vi "数据查询_仪器日志.vi"() -> ()   [LabVIEW 2016]
uses:
  <vilib>/Utility/miscctls.llb/LVRowAndColumnUnsignedTypeDef.ctl
  <vilib>/Utility/miscctls.llb/LVPointTypeDef.ctl
  <userlib>/_OpenG.lib/array/array.llb/Sort 2D Array (String)__ogtk.vi
panel:
  in  "序列号":string
  out "总共行数":i32
  in  "显示行数":i32=15
  in  "下拉列表":string(xcontrol)
  in  "导出":bool
  in  "查询":bool
  out "数据表":string[][](table)
  in  "结束日期":string="2050/01/01"
  in  "起始日期":string="2010/01/01"
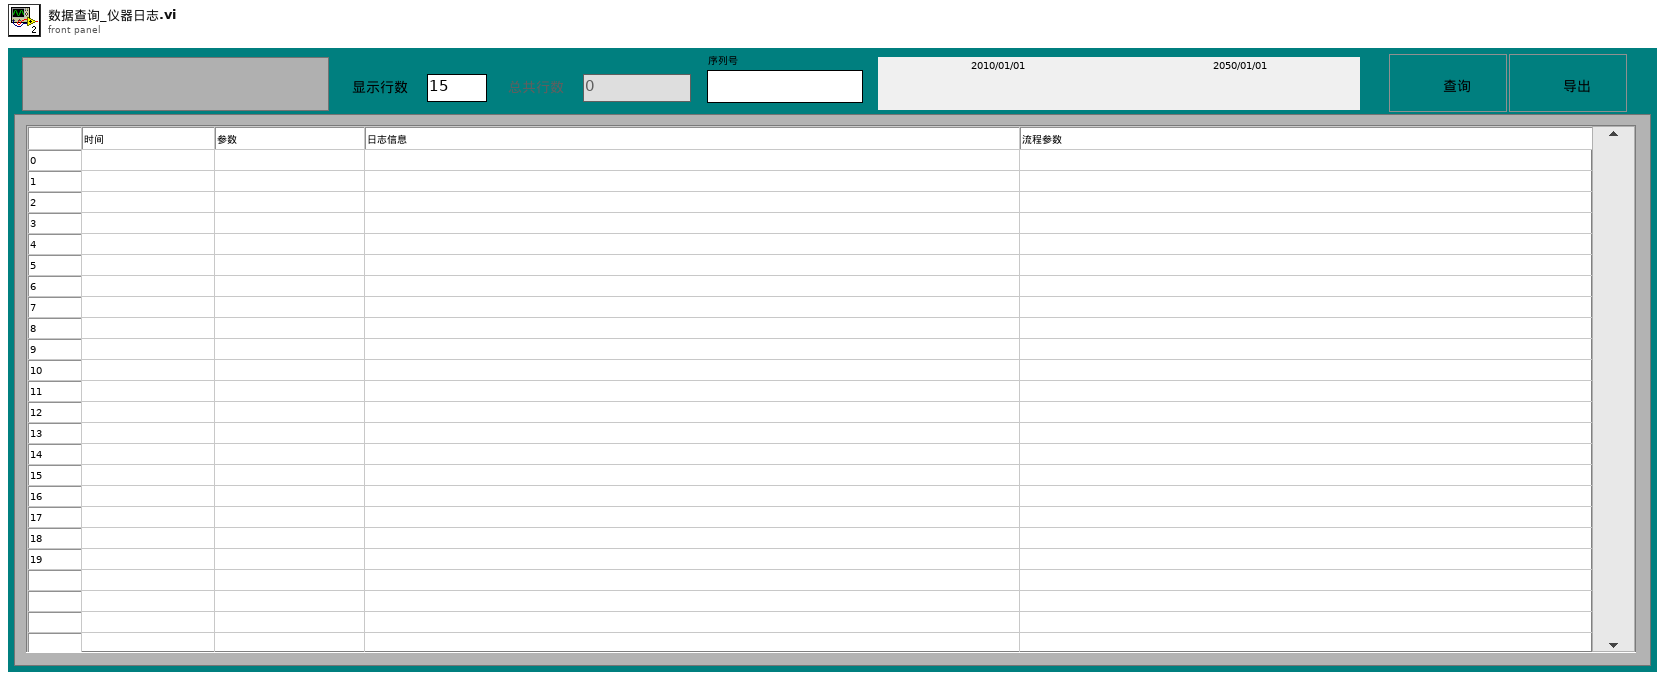
[diagram p1: front panel]
types:
  T1 = enum8{"Enabled", "Disabled", "Disabled and Grayed Out"}
  T2 = typedef "LVRowAndColumnUnsignedTypeDef.ctl" = cluster{"Row":u32, "Column":u32}
  T3 = typedef "LVPointTypeDef.ctl" = cluster{"Horizontal":i16, "Vertical":i16}
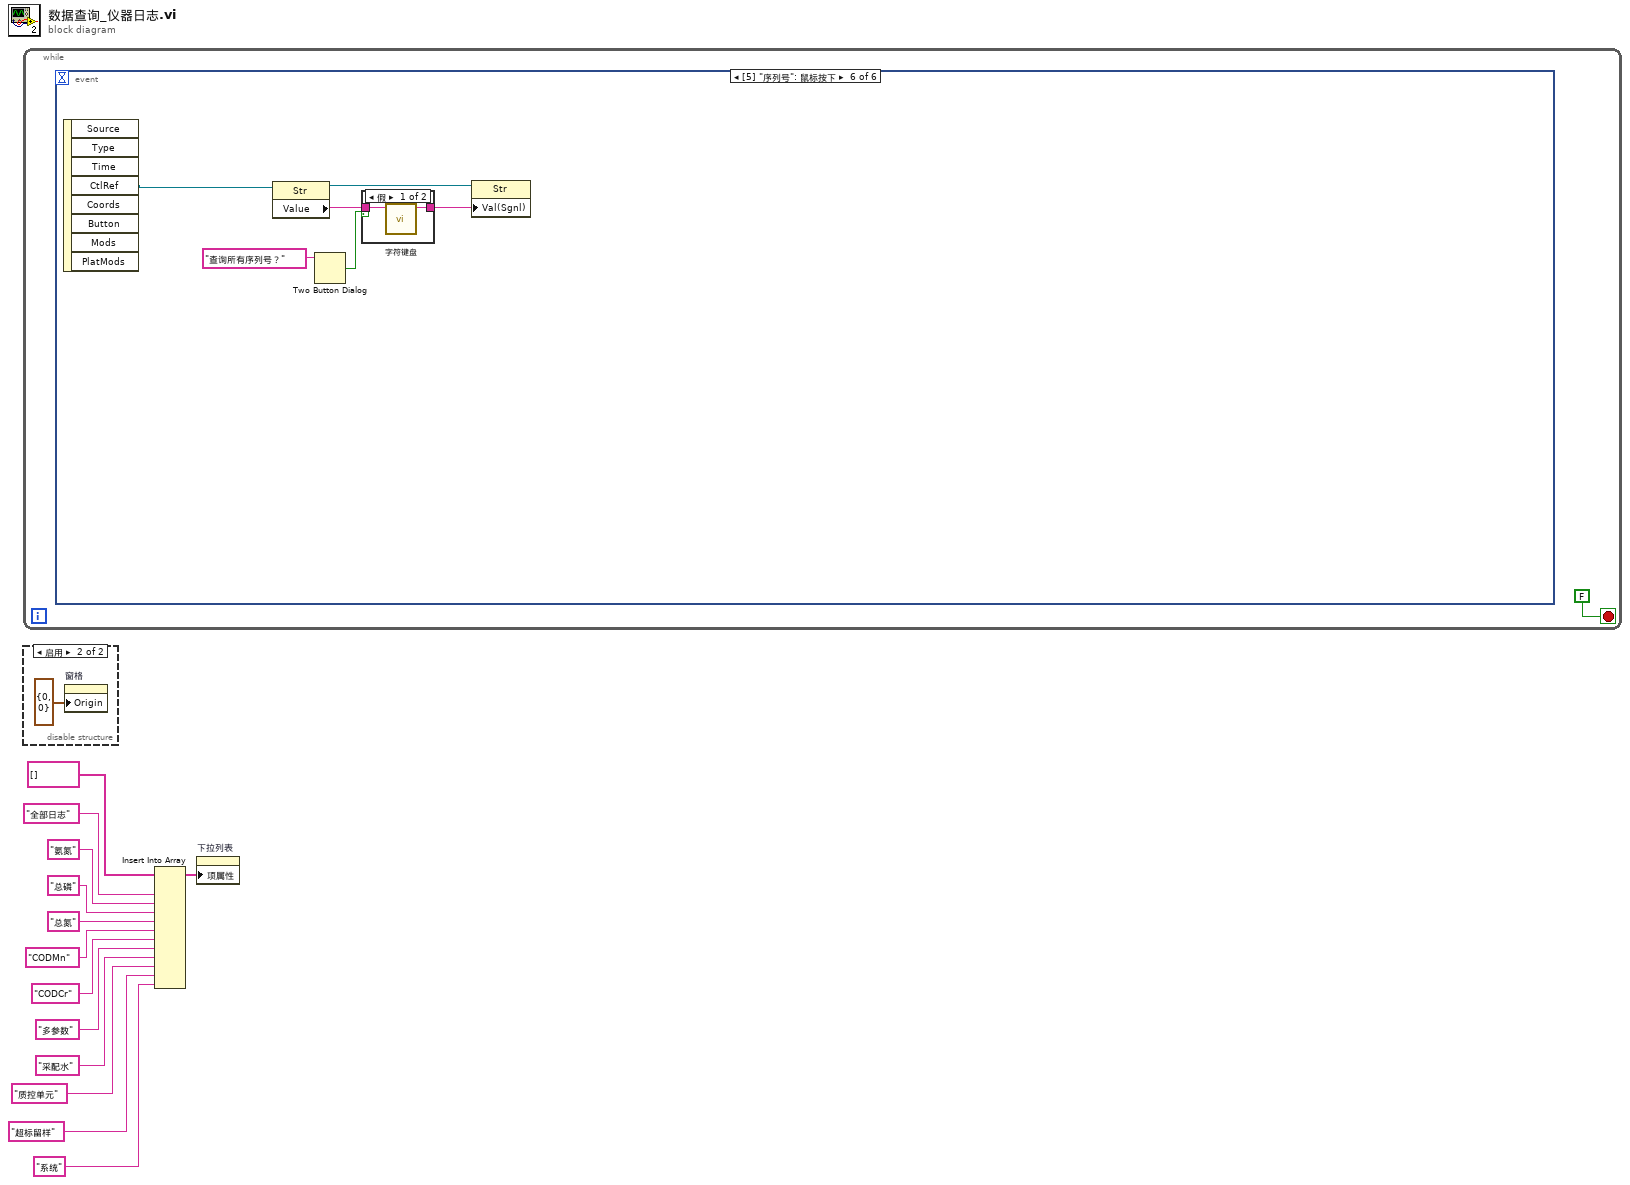
[diagram p0: block diagram]
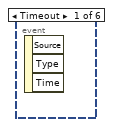
[diagram p2: hidden frame]
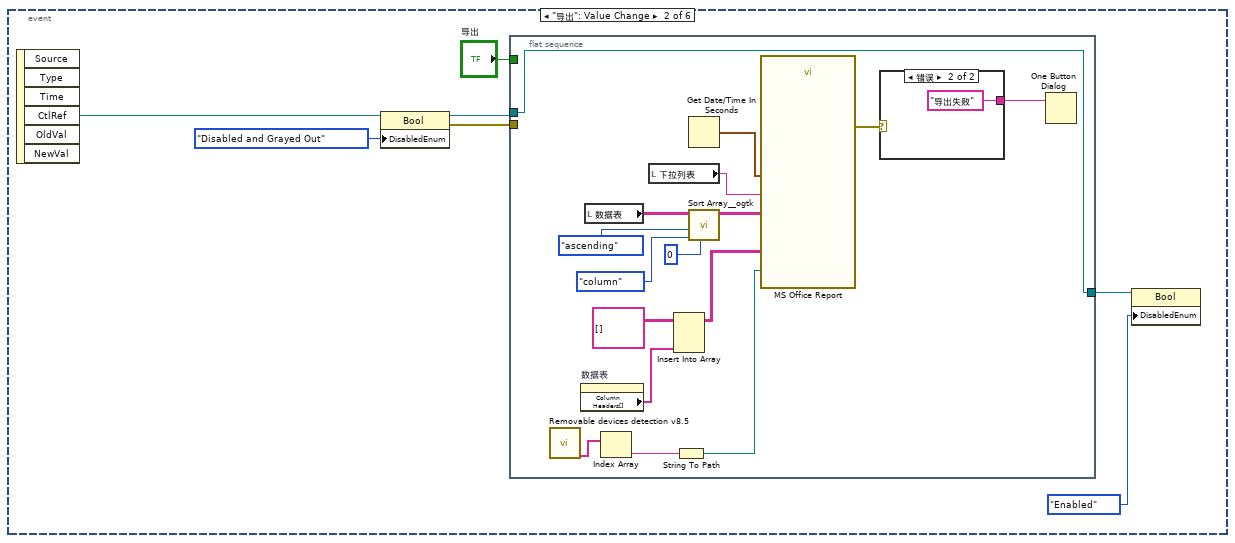
[diagram p3: hidden frame]
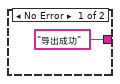
[diagram p4: hidden frame]
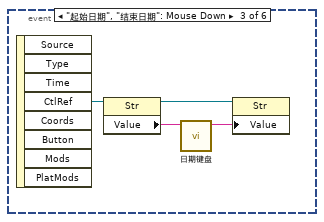
[diagram p5: hidden frame]
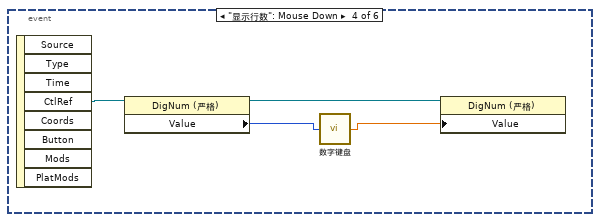
[diagram p6: hidden frame]
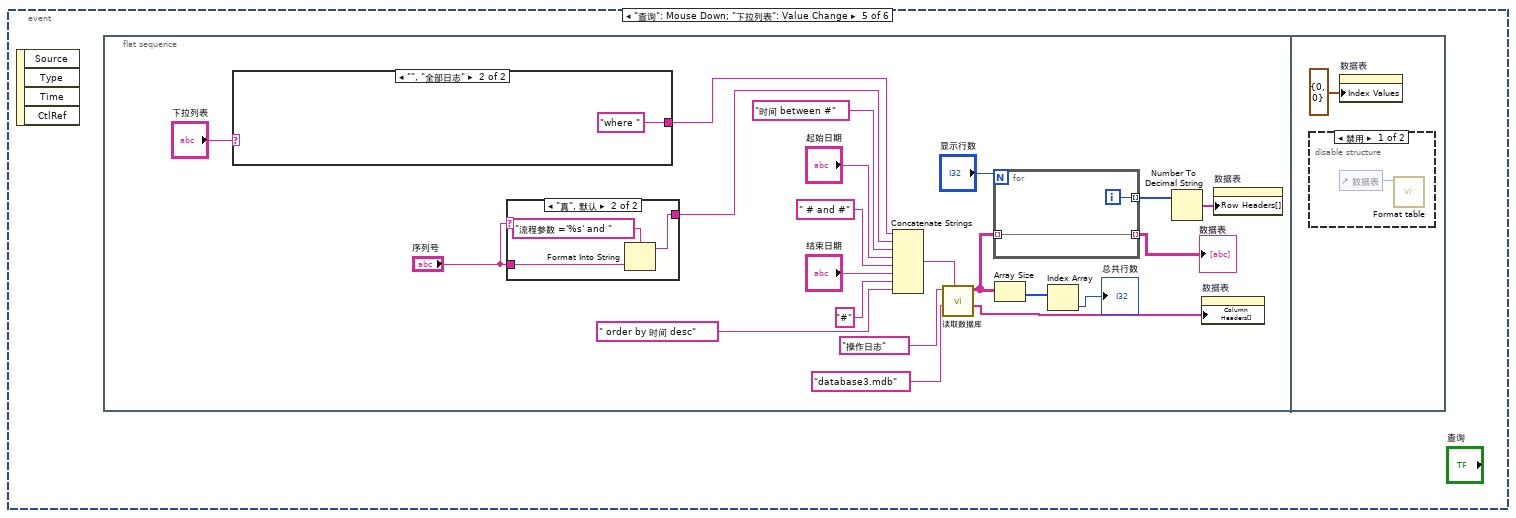
[diagram p7: hidden frame]
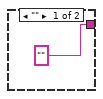
[diagram p8: hidden frame]
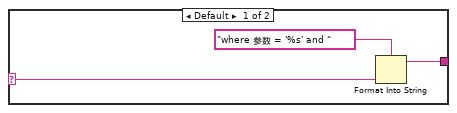
[diagram p9: hidden frame]
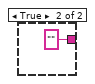
[diagram p11: hidden frame]
diagram:
  n1 = while {
    stop <- FALSE stop-if-true
    n2 = event shown="[5] \"序列号\": 鼠标按下" {
      selector: _ -> [_ _ _ _ _ _]
      dyn-events: _ -> [_ _ _ _ _ _]
      timeout: _ -> [_ _ _ _ _ _]
      event Timeout {
        n3 = event-data() -> ()  [unwired: 1 in, 3 out]
      }
      event "导出": Value Change {
        n4 = event-data() -> ("CtlRef"=w15:refnum<vi>)  [unwired: 1 in, 5 out]
        n5 = property class="Bool"(reference=w15, "DisabledEnum"=T1."Disabled and Grayed Out" ("禁用")) -> (reference out=w19:refnum<vi>, error out=w20:errorcluster)  [unwired: 1 in]
        n6 = flat-sequence {
          tunnel: w20 -> [_]
          tunnel: [w30] -> w18
          tunnel: w19 -> [w30]
          tunnel: "导出" -> [_]
          frame #0 {
            n7 = call "Removable devices detection v8.5.vi"() -> ("Removable"=w27:string[])  [unwired: 4 out]
            n8 = property on="数据表" class="Tbl (严格)"() -> ("Column Headers[]"=w22:string[])  [unwired: 2 in, 2 out]
            n9 = local read "数据表"() -> (w36:string[][])
            n10 = Index Array(array=w27) -> (element=w26:string)  [unwired: 1 in]
            n11 = local read "下拉列表"() -> (w31:string)
            n12 = Insert Into Array(array=string[][] [], new element=w22) -> (w23:string[][])  [unwired: 2 in]
            n13 = String To Path(string=w26) -> (path=w25:path)
            n14 = Get Date/Time In Seconds() -> (seconds since 1Jan1904=w37:timestamp)
            n15 = call-poly <userlib>:"Sort Array__ogtk.vi"("Column/Row to Sort By"=u32 0, "Sort By in"=enum16{"row", "column"}."column", "Order"=enum16{"ascending", "descending"}."ascending", "Array in"=w36) -> ("Sorted Array out"=w35:string[][])  [unwired: 4 in, 3 out]
            n16 = call "MS Office Report"("Path to Save Report"=w25, "导出日期"=w37, "监测参数"=w31, "数据输入"=w35, "字段定义"=w23) -> ("error out"=w29:errorcluster)  [unwired: 21 in, 1 out]
            n17 = case shown="错误" w29 {
              tunnel: ["导出成功" ("消息") "导出失败" ("消息")] -> w28
              frame No Error {
              }
              frame Error {
              }
            }
            n18 = One Button Dialog(message=w28) -> ()  [unwired: 1 in, 1 out]
          }
        }
        n19 = property class="Bool"(reference=w18, "DisabledEnum"=T1."Enabled" ("禁用")) -> ()  [unwired: 1 in, 2 out]
      }
      event "起始日期", "结束日期": Mouse Down {
        n20 = event-data() -> ("CtlRef"=w43:refnum<vi>)  [unwired: 1 in, 7 out]
        n21 = property class="Str"(reference=w43) -> (reference out=w41:refnum<vi>, "Value"=w42:string)  [unwired: 1 in, 1 out]
        n22 = call "日期键盘.vi"("原值"=w42) -> ("x+y"=w40:string)  [unwired: 10 in]
        n23 = property class="Str"(reference=w41, "Value"=w40) -> ()  [unwired: 1 in, 2 out]
      }
      event "显示行数": Mouse Down {
        n24 = event-data() -> ("CtlRef"=w47:refnum<vi>)  [unwired: 1 in, 7 out]
        n25 = property class="DigNum (严格)"(reference=w47) -> (reference out=w46:refnum<vi>, "Value"=w45:i32)  [unwired: 1 in, 1 out]
        n26 = call "数字键盘.vi"("OldNumber"=w45) -> ("NewNumber"=w44:sgl)
        n27 = property class="DigNum (严格)"(reference=w46, "Value"=w44) -> ()  [unwired: 1 in, 2 out]
      }
      event "查询": Mouse Down; "下拉列表": Value Change {
        n28 = event-data() -> ()  [unwired: 1 in, 4 out]
        n29 = flat-sequence {
          frame #0 {
            n30 = case shown="\"\", \"全部日志\"" "下拉列表" {
              selector: "下拉列表" -> [w73 _]
              tunnel: [w75 "where " ("condition")] -> w48
              frame Default {
                n31 = Format Into String(format string="where 参数 = '%s' and " ("condition"), w73) -> (resulting string=w75:string)  [unwired: 2 in, 1 out]
              }
              frame "", "全部日志" {
              }
            }
            n32 = case shown="\"真\", 默认" "序列号" {
              tunnel: "序列号" -> [_ w71]
              tunnel: ["" ("condition") w70] -> w50
              frame "" {
              }
              frame "真", Default {
                n33 = Format Into String(format string="流程参数 ='%s' and " ("condition"), w71) -> (resulting string=w70:string)  [unwired: 2 in, 1 out]
              }
            }
            n34 = Concatenate Strings(w48, w50, "时间 between #" ("condition"), "起始日期", " # and #" ("condition"), "结束日期", "#" ("condition"), " order by 时间 desc" ("字符串")) -> (w67:string)
            n35 = call "读取数据库.vi"("condition"=w67, "database"="database3.mdb", "组合框"="操作日志") -> ("columns"=w63:string[], "表格"=w54:string[][])  [unwired: 5 in, 2 out]
            n36 = for {
              N: "显示行数" -> [_]
              tunnel: w54 -> [w77] mode=indexing
              tunnel: [w78] -> w60 mode=indexing
              tunnel: [w77] -> w56 mode=indexing
              i -> [w78]
            }
            "数据表" <- w56
            n37 = Array Size(array=w54) -> (size(s)=w53:i32[])
            n38 = Index Array(array=w53) -> (element=→"总共行数":i32)  [unwired: 1 in]
            n39 = Number To Decimal String(number=w60) -> (decimal integer string=w59:string[])  [unwired: 1 in]
            n40 = property on="数据表" class="Tbl (严格)"("Column Headers[]"=w63) -> ()  [unwired: 2 in, 2 out]
            n41 = property on="数据表" class="Tbl (严格)"("Row Headers[]"=w59) -> ()  [unwired: 2 in, 2 out]
          }
          frame #1 {
            n42 = disable-structure shown="禁用" {
              frame Disabled {
                n43 = control-ref of="数据表"() -> (w80:refnum<vi>)
                n44 = call "Format table.vi"("Table输入"=w80) -> ()  [unwired: 11 in]
              }
              frame Enabled {
              }
            }
            n45 = property on="数据表" class="Tbl (严格)"("Index Values"=T2 {"Row"=0, "Column"=0} ("索引值")) -> ()  [unwired: 2 in, 2 out]
          }
        }
      }
      event "序列号": Mouse Down {
        n46 = event-data() -> ("CtlRef"=w81:refnum<vi>)  [unwired: 1 in, 7 out]
        n47 = property class="Str"(reference=w81) -> (reference out=w85:refnum<vi>, "Value"=w86:string)  [unwired: 1 in, 1 out]
        n48 = Two Button Dialog(message="查询所有序列号？" ("消息")) -> (T button?=w82:bool)  [unwired: 2 in]
        n49 = case shown="假" w82 {
          tunnel: w86 -> [w88 _]
          tunnel: [w87 "" ("x+y")] -> w84
          frame False {
            n50 = call "字符键盘.vi"("原值"=w88) -> ("x+y"=w87:string)  [unwired: 10 in]
          }
          frame True {
          }
        }
        n51 = property class="Str"(reference=w85, "Val(Sgnl)"=w84) -> ()  [unwired: 1 in, 2 out]
      }
    }
  }
  n52 = disable-structure shown="启用" {
    frame Disabled {
    }
    frame Enabled {
      n53 = property on="窗格" class="Pane"("Origin"=T3 {"Horizontal"=0, "Vertical"=0} ("原点")) -> ()  [unwired: 2 in, 2 out]
    }
  }
  n54 = Insert Into Array(array=string[] [], new element #1="全部日志" ("新元素/子数组"), new element #2="氨氮" ("新元素/子数组"), new element #3="总磷" ("新元素/子数组"), new element #4="总氮" ("新元素/子数组"), new element #5="CODMn" ("新元素/子数组"), new element #6="CODCr" ("新元素/子数组"), new element #7="多参数" ("新元素/子数组"), new element #8="采配水" ("新元素/子数组"), new element #9="质控单元" ("新元素/子数组"), new element #10="超标留样" ("新元素/子数组"), new element #11="系统" ("新元素/子数组")) -> (w4:string[])  [unwired: 1 in]
  n55 = property on="下拉列表" class="下拉列表 (严格)"("项属性"=w4) -> ()  [unwired: 2 in, 2 out]
